vi "PFI-28000-System_Get Test.vi"(8 "error in (no error)":errorcluster, 11 "PFI-28000-System in":refnum<class "PFI-28000-System.lvclass">) -> (0 "error out":errorcluster, 2 "Enabled":bool, 3 "PFI-28000-System out":refnum<class "PFI-28000-System.lvclass">)   [LabVIEW 2017, in "PFI-28000-System.lvclass"]
uses:
  PFI-28000-System.lvclass
  Utilities/PFI-28000-Utils.lvlib
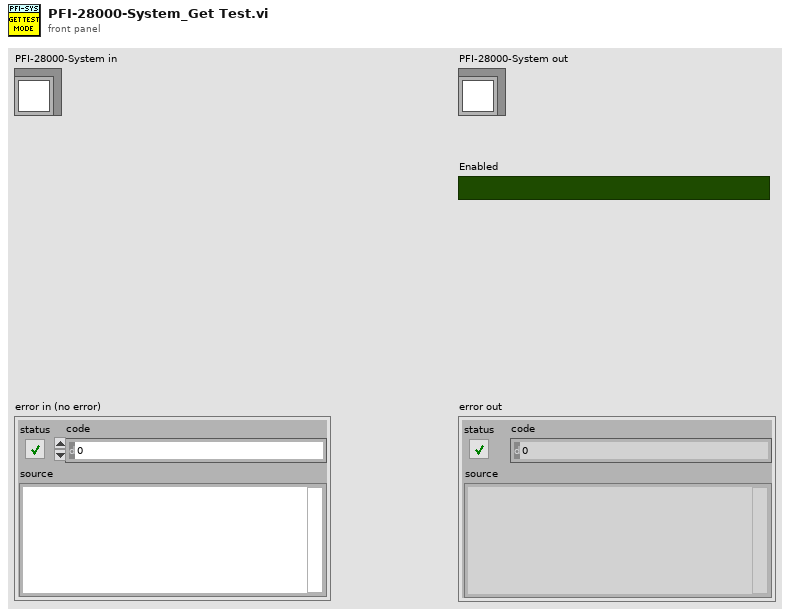
[diagram p1: front panel]
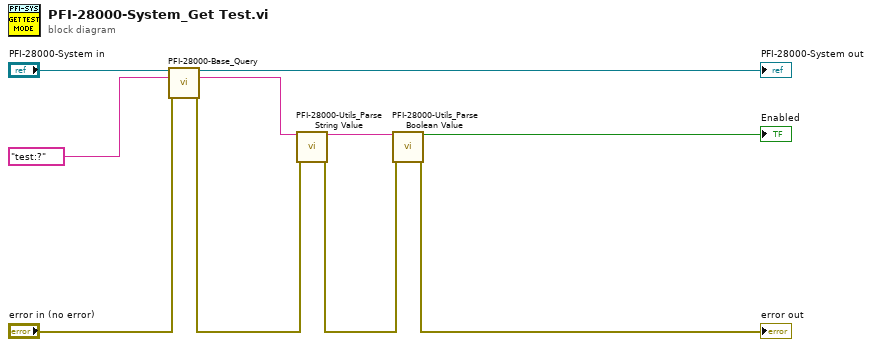
[diagram p0: block diagram]
diagram:
  n1 = call-dynamic "PFI-28000-Base_Query.vi"("PFI-28000-Base in"="PFI-28000-System in", "Command"="test:?", "error in (no error)"="error in (no error)") -> ("PFI-28000-Base out"=→"PFI-28000-System out":refnum<class "PFI-28000-System.lvclass">, "Response"=w1:string, "error out"=w3:errorcluster)  [unwired: 9 in, 1 out]
  n2 = call "PFI-28000-Utils_Parse String Value.vi"("String"=w1, "error in (no error)"=w3) -> ("String Value"=w8:string, "error out"=w7:errorcluster)  [unwired: 11 in, 1 out]
  n3 = call "PFI-28000-Utils_Parse Boolean Value.vi"("String"=w8, "error in (no error)"=w7) -> ("Value"=→"Enabled":bool, "error out"=→"error out":errorcluster)  [unwired: 12 in]
